vi "检测结果.vi"() -> ()   [LabVIEW 2020]
panel:
  in  "曲线":refnum<vi>
  in  "零位油压":string
  in  "自由间隙":string
  in  "空载扭矩":string
  in  "最大扭矩":string
  in  "最大油压":string
  in  "合格状态":string
  in  "总圈数":string
  in  "外泄露":string
  in  "回正扭矩":string
  in  "功能试验":string
  in  "内泄露":string
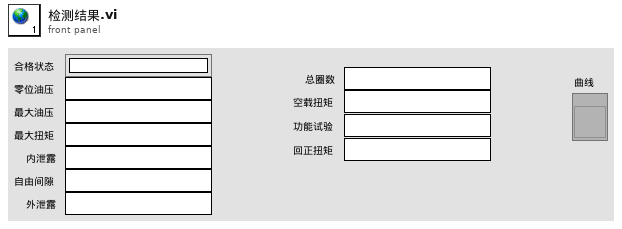
[diagram p1: front panel]
diagram:
